vi "GetEnumValueAndPosition__slk_mt.vi"(7 "create enum configure":T1, 8 "error in (no error)":errorcluster, 11 "selection list":refnum<vi>[](array[refnum])) -> (0 "error out":errorcluster, 2 "position":cluster{"Left":i32, "Top":i32}, 3 "values":string[](array[string]), 4 "not found?":bool)   [LabVIEW 2013, in "Lazyboots Menu Tool.lvlib"]
doc: "Returns enum value and position."
uses:
  Library/Lazyboots Menu Tool.lvlib
  <vilib>/Utility/miscctls.llb/LVPositionTypeDef.ctl
  TypeDef/TypeDef_CreateEnumConfigure__slk_mt.ctl
panel:
  # "GetEnumValueAndPosition__slk_mt.vi\nReturns enum value and position.\n\nNOTICE -- YOU MUST LEAVE THIS NOTICE IN PLACE.\n\nCopyright (c) 2011, LIANG LIU Shawn.Liu.cn@gmail.com\nAll rights reserved.\n\nRedistribution and use in source and binary forms, with or without modification, are permitted provided that the following conditions are met:\n-Redistributions of source code must retain the above copyright notice, this list of conditions and the following disclaimer.\n-Redistributions in binary form must reproduce the above copyright notice, this list of conditions and the following disclaimer in the documentation and/or other materials provided with the distribution.\n-Neither the name of the eLp nor the names of its contributors may be used to endorse or promote products derived from this software without specific prior written permission.\n\nTHIS SOFTWARE IS PROVIDED BY THE COPYRIGHT HOLDERS AND CONTRIBUTORS \"AS IS\" AND ANY EXPRESS OR IMPLIED WARRANTIES, INCLUDING, BUT NOT LIMITED TO, THE IMPLIED WARRANTIES OF MERCHANTABILITY AND FITNESS FOR A PARTICULAR PURPOSE ARE DISCLAIMED. IN NO EVENT SHALL THE COPYRIGHT HOLDER OR CONTRIBUTORS BE LIABLE FOR ANY DIRECT, INDIRECT, INCIDENTAL, SPECIAL, EXEMPLARY, OR CONSEQUENTIAL DAMAGES (INCLUDING, BUT NOT LIMITED TO, PROCUREMENT OF SUBSTITUTE GOODS OR SERVICES; LOSS OF USE, DATA, OR PROFITS; OR BUSINESS INTERRUPTION) HOWEVER CAUSED AND ON ANY THEORY OF LIABILITY, WHETHER IN CONTRACT, STRICT LIABILITY, OR TORT (INCLUDING NEGLIGENCE OR OTHERWISE) ARISING IN ANY WAY OUT OF THE USE OF THIS SOFTWARE, EVEN IF ADVISED OF THE POSSIBILITY OF SUCH DAMAGE."
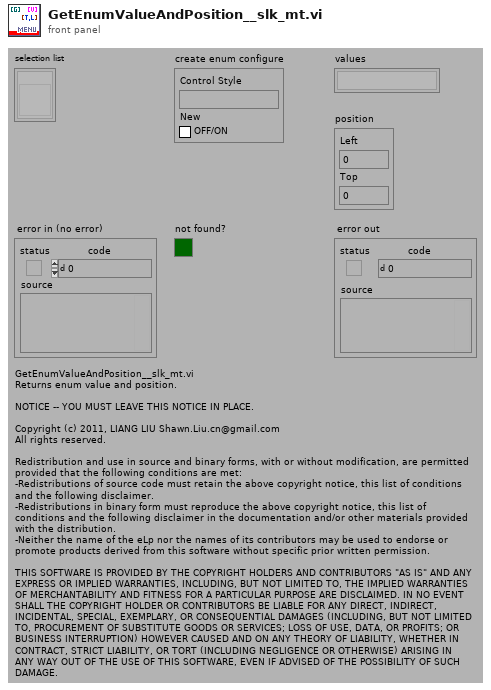
[diagram p1: front panel]
types:
  T1 = typedef "Lazyboots Menu Tool.lvlib/TypeDef_CreateEnumConfigure__slk_mt.ctl" = cluster{"Control Style":string, "New":bool}
  T2 = typedef "LVPositionTypeDef.ctl" = cluster{"Left":i32, "Top":i32}
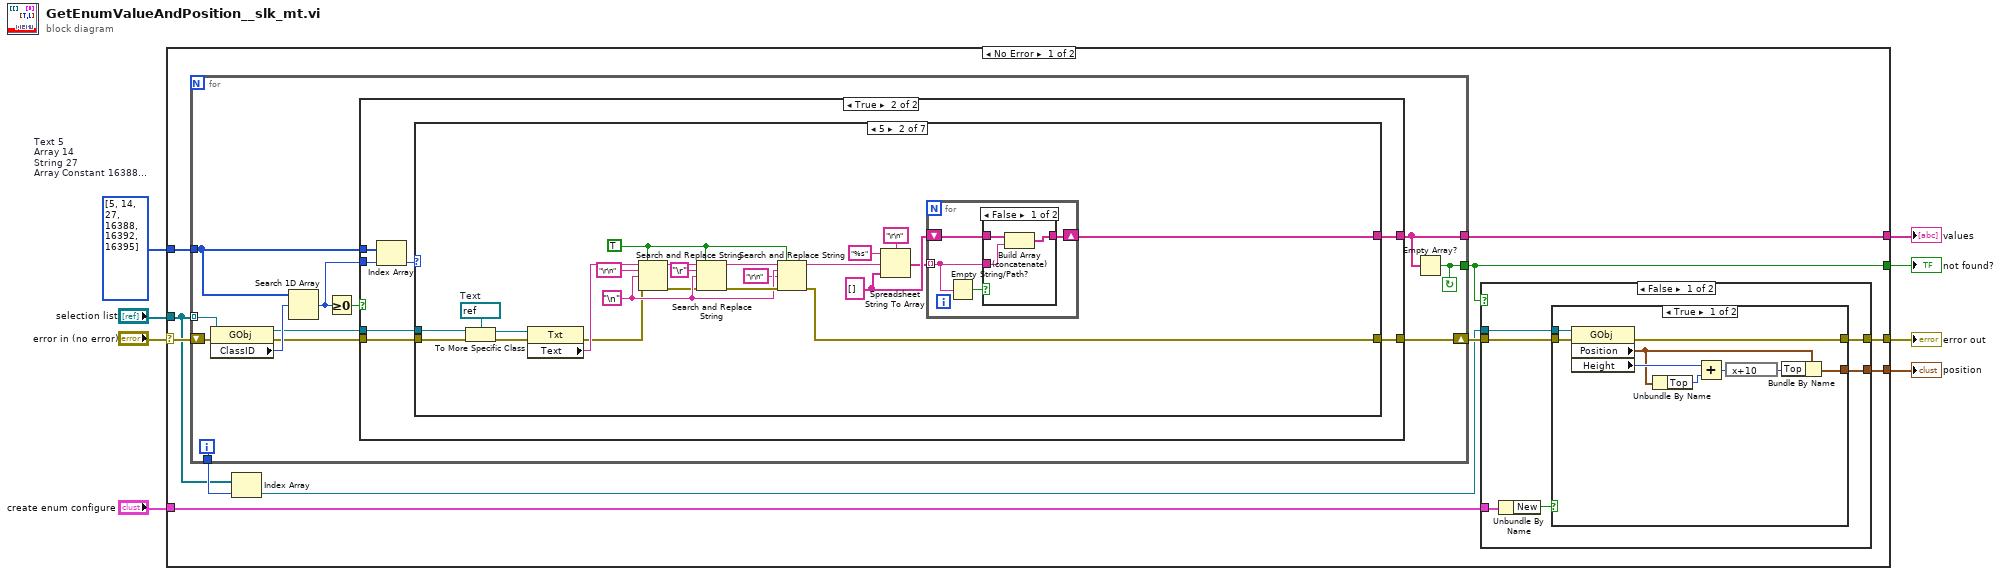
[diagram p0: block diagram]
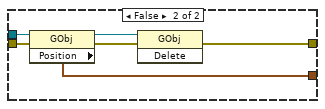
[diagram p2: hidden frame]
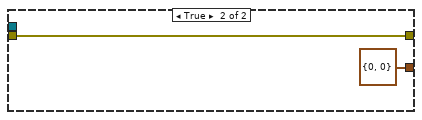
[diagram p3: hidden frame]
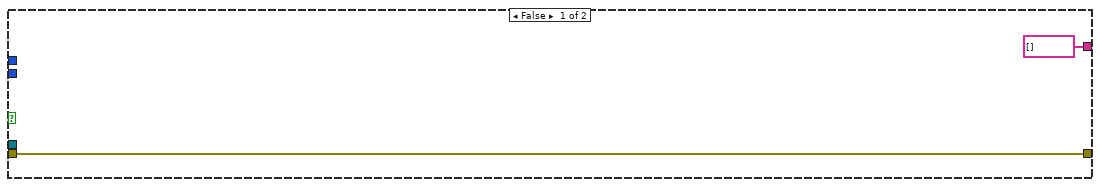
[diagram p4: hidden frame]
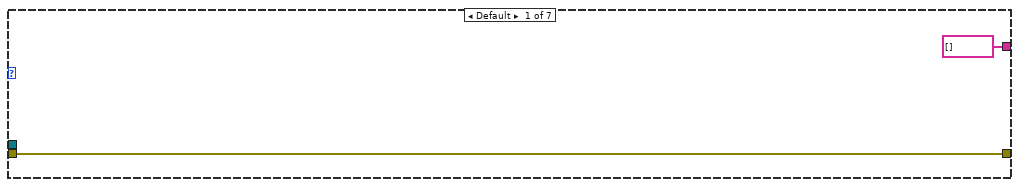
[diagram p5: hidden frame]
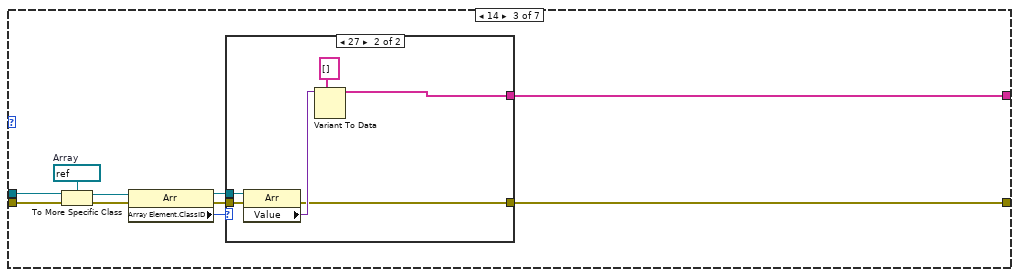
[diagram p7: hidden frame]
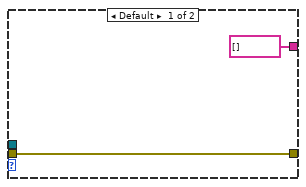
[diagram p8: hidden frame]
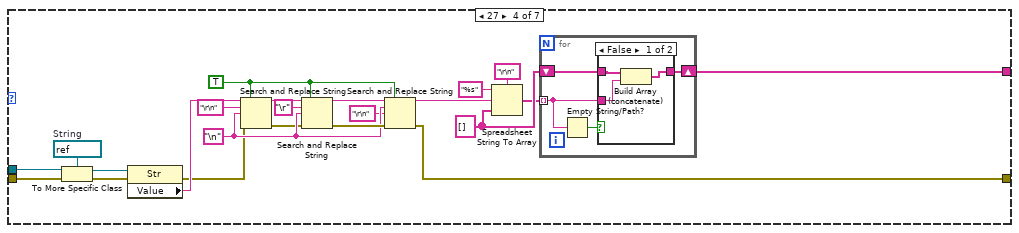
[diagram p9: hidden frame]
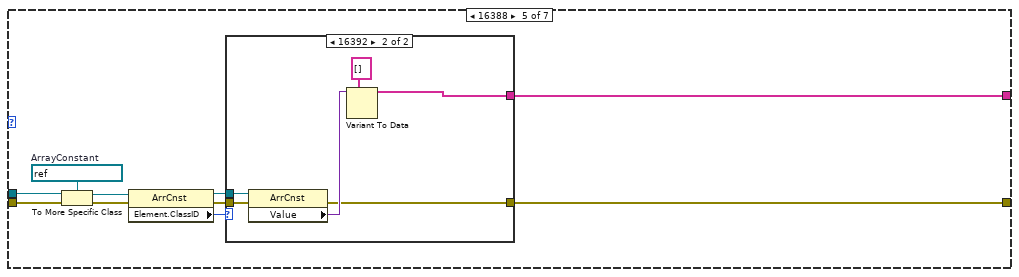
[diagram p11: hidden frame]
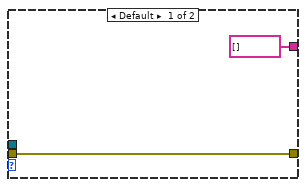
[diagram p12: hidden frame]
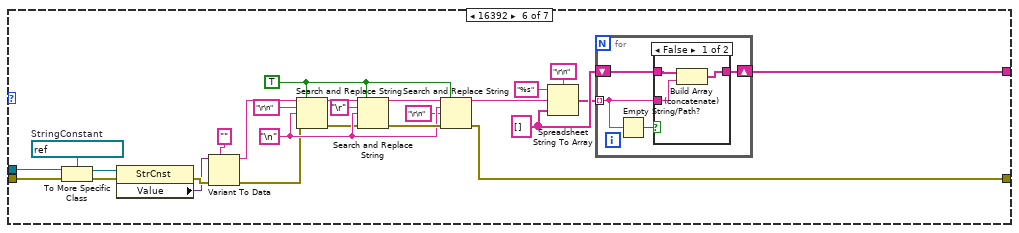
[diagram p13: hidden frame]
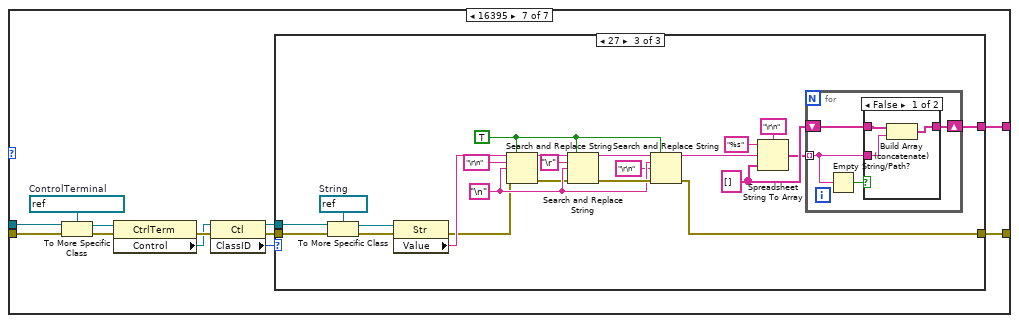
[diagram p15: hidden frame]
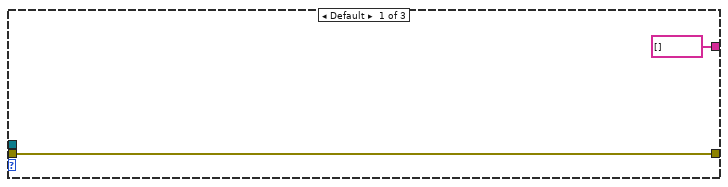
[diagram p16: hidden frame]
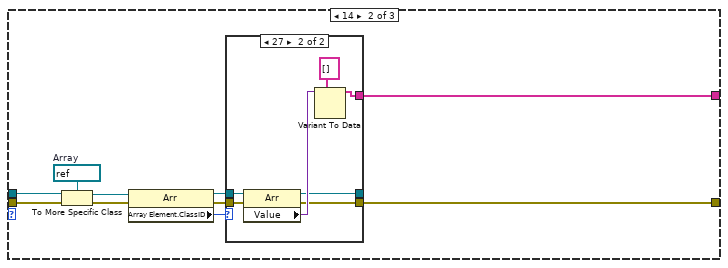
[diagram p17: hidden frame]
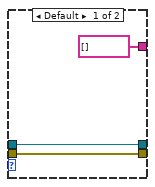
[diagram p18: hidden frame]
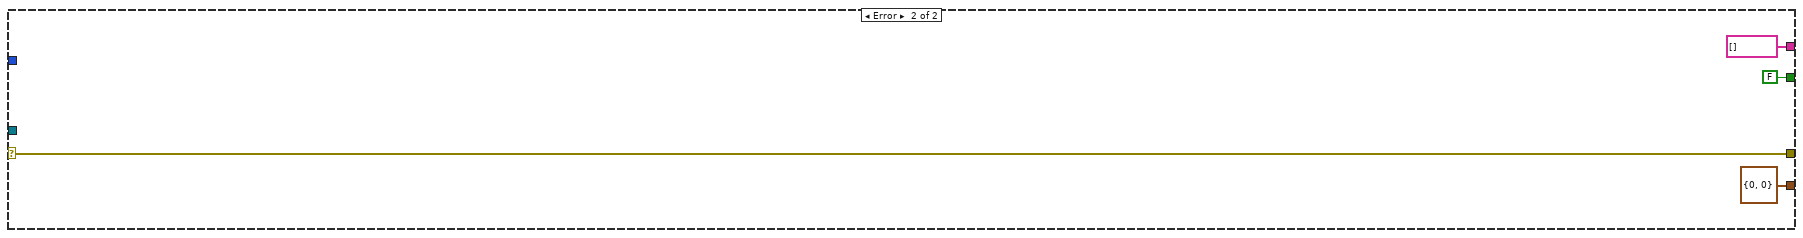
[diagram p20: hidden frame]
diagram:
  w8 = u32[] [5, 14, 27, 16388, 16392, 16395]  # Text 5 Array 14 String 27 Array Constant 16388 String Constant 16392 Control Terminal 16395
  n1 = case shown="No Error" "error in (no error)" {
    selector: "error in (no error)" -> [w17 w266]
    tunnel: w8 -> [w19 _]
    tunnel: [w18 string[] []] -> w7
    tunnel: "selection list" -> [w14 _]
    tunnel: [w12 FALSE ("empty?")] -> w4
    tunnel: [w11 w266] -> w3
    tunnel: [w10 T2 {"Left"=0, "Top"=0} ("Position")] -> w2
    tunnel: "create enum configure" -> [w9 _]
    frame No Error {
      n2 = for {
        tunnel: w19 -> [w53]
        tunnel: [w47] -> w18
        tunnel: w14 -> [w48] mode=indexing
        tunnel: [w46] -> w12
        shift-right: [w45] -> w16
        shift-left: w17 -> [w44]
        tunnel: [w43] -> w15
        i -> [w43]
        stop <- w46 continue-if-true
        n3 = property class="GObj"(reference=w48, error in=w44) -> (reference out=w50:refnum<vi>, error out=w49:errorcluster, "ClassID"=w54:u32)
        n4 = Search 1D Array(1D array=w53, element=w54) -> (index of element=w51:i32)  [unwired: 1 in]
        n5 = Greater Or Equal To 0?(x=w51) -> (x >= 0?=w52:bool)
        n6 = case shown="True" w52 {
          tunnel: w53 -> [_ w63]
          tunnel: w51 -> [_ w62]
          tunnel: w50 -> [_ w59]
          tunnel: w49 -> [w56 w60]
          tunnel: [w56 w57] -> w45
          tunnel: [string[] [] w58] -> w47
          frame False {
          }
          frame True {
            n7 = Index Array(array=w63, index=w62) -> (element=w61:u32)
            n8 = case shown="5" w61 {
              tunnel: w60 -> [w64 w70 w105 w119 w154 w172 w207]
              tunnel: w59 -> [_ w69 w104 w118 w153 w171 w206]
              tunnel: [w64 w67 w99 w116 w148 w169 w200] -> w57
              tunnel: [string[] [] w66 w100 w115 w149 w168 w199] -> w58
              frame Default {
              }
              frame 5 {
                w82 = string[] []
                w86 = "\n" ("search string")
                w88 = TRUE ("replace all? (F)")
                w71 = refnum<vi> refnum  # Text
                n9 = To More Specific Class(target class=w71, reference=w69, error in=w70) -> (specific class reference=w73:refnum<vi>, error out=w72:errorcluster)
                n10 = property class="Txt"(reference=w73, error in=w72) -> (error out=w68:errorcluster, "Text"=w77:string)  [unwired: 1 out]
                n11 = Search and Replace String(replace all?=w88, input string=w77, search string="\r\n", replace string=w86, error in=w68) -> (result string=w76:string, error out=w78:errorcluster)  [unwired: 5 out]
                n12 = Search and Replace String(replace all?=w88, input string=w76, search string="\r", replace string=w86, error in=w78) -> (result string=w85:string, error out=w87:errorcluster)  [unwired: 5 out]
                n13 = Search and Replace String(replace all?=w88, input string=w85, search string=w86, replace string="\r\n" ("replace string (\"\")"), error in=w87) -> (result string=w84:string, error out=w67:errorcluster)  [unwired: 3 in, 2 out]
                n14 = Spreadsheet String To Array(delimiter (Tab)="\r\n" ("search string"), format string="%s", spreadsheet string=w84, array type (2D Dbl)=w82) -> (array=w81:string[])
                n15 = for {
                  tunnel: w81 -> [w91] mode=indexing
                  shift-right: [w89] -> w66
                  shift-left: w82 -> [w90]
                  n16 = Empty String/Path?(string/path=w91) -> (empty?=w92:bool)
                  n17 = case shown="False" w92 {
                    tunnel: w91 -> [w93 _]
                    tunnel: w90 -> [w95 w96]
                    tunnel: [w94 w96] -> w89
                    frame False {
                      n18 = Build Array (concatenate)(w95, w93) -> (w94:string[])
                    }
                    frame True {
                    }
                  }
                }
              }
              frame 14 {
                w106 = refnum<vi> refnum  # Array
                n19 = To More Specific Class(target class=w106, reference=w104, error in=w105) -> (specific class reference=w101:refnum<vi>, error out=w102:errorcluster)
                n20 = property class="Arr"(reference=w101, error in=w102) -> (reference out=w98:refnum<vi>, error out=w97:errorcluster, "Array Element.ClassID"=w103:u32)
                n21 = case shown="27" w103 {
                  tunnel: [w108 w111] -> w99
                  tunnel: [string[] [] w112] -> w100
                  tunnel: w98 -> [_ w110]
                  tunnel: w97 -> [w108 w109]
                  frame Default {
                  }
                  frame 27 {
                    n22 = property class="Arr"(reference=w110, error in=w109) -> (error out=w111:errorcluster, "Value"=w114:variant)  [unwired: 1 out]
                    n23 = Variant To Data(type=string[] [], Variant=w114) -> (data=w112:string[])  [unwired: 1 in, 1 out]
                  }
                }
              }
              frame 27 {
                w131 = string[] []
                w135 = "\n" ("search string")
                w137 = TRUE ("replace all? (F)")
                w120 = refnum<vi> refnum  # String
                n24 = To More Specific Class(target class=w120, reference=w118, error in=w119) -> (specific class reference=w122:refnum<vi>, error out=w121:errorcluster)
                n25 = property class="Str"(reference=w122, error in=w121) -> (error out=w117:errorcluster, "Value"=w126:string)  [unwired: 1 out]
                n26 = Search and Replace String(replace all?=w137, input string=w126, search string="\r\n", replace string=w135, error in=w117) -> (result string=w125:string, error out=w127:errorcluster)  [unwired: 5 out]
                n27 = Search and Replace String(replace all?=w137, input string=w125, search string="\r", replace string=w135, error in=w127) -> (result string=w134:string, error out=w136:errorcluster)  [unwired: 5 out]
                n28 = Search and Replace String(replace all?=w137, input string=w134, search string=w135, replace string="\r\n" ("replace string (\"\")"), error in=w136) -> (result string=w133:string, error out=w116:errorcluster)  [unwired: 3 in, 2 out]
                n29 = Spreadsheet String To Array(delimiter (Tab)="\r\n" ("search string"), format string="%s", spreadsheet string=w133, array type (2D Dbl)=w131) -> (array=w130:string[])
                n30 = for {
                  tunnel: w130 -> [w140] mode=indexing
                  shift-right: [w138] -> w115
                  shift-left: w131 -> [w139]
                  n31 = Empty String/Path?(string/path=w140) -> (empty?=w141:bool)
                  n32 = case shown="False" w141 {
                    tunnel: w140 -> [w142 _]
                    tunnel: w139 -> [w144 w145]
                    tunnel: [w143 w145] -> w138
                    frame False {
                      n33 = Build Array (concatenate)(w144, w142) -> (w143:string[])
                    }
                    frame True {
                    }
                  }
                }
              }
              frame 16388 {
                w155 = refnum<vi> refnum  # ArrayConstant
                n34 = To More Specific Class(target class=w155, reference=w153, error in=w154) -> (specific class reference=w150:refnum<vi>, error out=w151:errorcluster)
                n35 = property class="ArrCnst"(reference=w150, error in=w151) -> (reference out=w147:refnum<vi>, error out=w146:errorcluster, "Element.ClassID"=w152:u32)
                n36 = case shown="16392" w152 {
                  tunnel: [w157 w160] -> w148
                  tunnel: [string[] [] w161] -> w149
                  tunnel: w147 -> [_ w159]
                  tunnel: w146 -> [w157 w158]
                  frame Default {
                  }
                  frame 16392 {
                    n37 = property class="ArrCnst"(reference=w159, error in=w158) -> (error out=w160:errorcluster, "Value"=w163:variant)  [unwired: 1 out]
                    n38 = Variant To Data(type=string[] [], Variant=w163) -> (data=w161:string[])  [unwired: 1 in, 1 out]
                  }
                }
              }
              frame 16392 {
                w183 = string[] []
                w187 = "\n" ("search string")
                w189 = TRUE ("replace all? (F)")
                w173 = refnum<vi> refnum  # StringConstant
                n39 = To More Specific Class(target class=w173, reference=w171, error in=w172) -> (specific class reference=w175:refnum<vi>, error out=w174:errorcluster)
                n40 = property class="StrCnst"(reference=w175, error in=w174) -> (error out=w170:errorcluster, "Value"=w166:variant)  [unwired: 1 out]
                n41 = Variant To Data(error in=w170, type="", Variant=w166) -> (data=w165:string, error out=w167:errorcluster)
                n42 = Search and Replace String(replace all?=w189, input string=w165, search string="\r\n", replace string=w187, error in=w167) -> (result string=w178:string, error out=w179:errorcluster)  [unwired: 5 out]
                n43 = Search and Replace String(replace all?=w189, input string=w178, search string="\r", replace string=w187, error in=w179) -> (result string=w186:string, error out=w188:errorcluster)  [unwired: 5 out]
                n44 = Search and Replace String(replace all?=w189, input string=w186, search string=w187, replace string="\r\n" ("replace string (\"\")"), error in=w188) -> (result string=w185:string, error out=w169:errorcluster)  [unwired: 3 in, 2 out]
                n45 = Spreadsheet String To Array(delimiter (Tab)="\r\n" ("search string"), format string="%s", spreadsheet string=w185, array type (2D Dbl)=w183) -> (array=w182:string[])
                n46 = for {
                  tunnel: w182 -> [w192] mode=indexing
                  shift-right: [w190] -> w168
                  shift-left: w183 -> [w191]
                  n47 = Empty String/Path?(string/path=w192) -> (empty?=w193:bool)
                  n48 = case shown="False" w193 {
                    tunnel: w192 -> [w194 _]
                    tunnel: w191 -> [w196 w197]
                    tunnel: [w195 w197] -> w190
                    frame False {
                      n49 = Build Array (concatenate)(w196, w194) -> (w195:string[])
                    }
                    frame True {
                    }
                  }
                }
              }
              frame 16395 {
                w208 = refnum<vi> refnum  # ControlTerminal
                n50 = To More Specific Class(target class=w208, reference=w206, error in=w207) -> (specific class reference=w198:refnum<vi>, error out=w209:errorcluster)
                n51 = property class="CtrlTerm"(reference=w198, error in=w209) -> (error out=w205:errorcluster, "Control"=w204:refnum<vi>)  [unwired: 1 out]
                n52 = property class="Ctl"(reference=w204, error in=w205) -> (reference out=w202:refnum<vi>, error out=w203:errorcluster, "ClassID"=w201:u32)
                n53 = case shown="27" w201 {
                  tunnel: w203 -> [w210 w220 w236]
                  tunnel: w202 -> [_ w219 w235]
                  tunnel: [w210 w214 w233] -> w200
                  tunnel: [string[] [] w215 w232] -> w199
                  frame Default {
                  }
                  frame 14 {
                    w221 = refnum<vi> refnum  # Array
                    n54 = To More Specific Class(target class=w221, reference=w219, error in=w220) -> (specific class reference=w216:refnum<vi>, error out=w217:errorcluster)
                    n55 = property class="Arr"(reference=w216, error in=w217) -> (reference out=w213:refnum<vi>, error out=w212:errorcluster, "Array Element.ClassID"=w218:u32)
                    n56 = case shown="27" w218 {
                      tunnel: [w224 w228] -> w214
                      tunnel: [string[] [] w229] -> w215
                      tunnel: [w223 w227] -> _
                      tunnel: w213 -> [w223 w226]
                      tunnel: w212 -> [w224 w225]
                      frame Default {
                      }
                      frame 27 {
                        n57 = property class="Arr"(reference=w226, error in=w225) -> (reference out=w227:refnum<vi>, error out=w228:errorcluster, "Value"=w231:variant)
                        n58 = Variant To Data(type=string[] [], Variant=w231) -> (data=w229:string[])  [unwired: 1 in, 1 out]
                      }
                    }
                  }
                  frame 27 {
                    w248 = string[] []
                    w252 = "\n" ("search string")
                    w254 = TRUE ("replace all? (F)")
                    w237 = refnum<vi> refnum  # String
                    n59 = To More Specific Class(target class=w237, reference=w235, error in=w236) -> (specific class reference=w239:refnum<vi>, error out=w238:errorcluster)
                    n60 = property class="Str"(reference=w239, error in=w238) -> (error out=w234:errorcluster, "Value"=w243:string)  [unwired: 1 out]
                    n61 = Search and Replace String(replace all?=w254, input string=w243, search string="\r\n", replace string=w252, error in=w234) -> (result string=w242:string, error out=w244:errorcluster)  [unwired: 5 out]
                    n62 = Search and Replace String(replace all?=w254, input string=w242, search string="\r", replace string=w252, error in=w244) -> (result string=w251:string, error out=w253:errorcluster)  [unwired: 5 out]
                    n63 = Search and Replace String(replace all?=w254, input string=w251, search string=w252, replace string="\r\n" ("replace string (\"\")"), error in=w253) -> (result string=w250:string, error out=w233:errorcluster)  [unwired: 3 in, 2 out]
                    n64 = Spreadsheet String To Array(delimiter (Tab)="\r\n" ("search string"), format string="%s", spreadsheet string=w250, array type (2D Dbl)=w248) -> (array=w247:string[])
                    n65 = for {
                      tunnel: w247 -> [w257] mode=indexing
                      shift-right: [w255] -> w232
                      shift-left: w248 -> [w256]
                      n66 = Empty String/Path?(string/path=w257) -> (empty?=w258:bool)
                      n67 = case shown="False" w258 {
                        tunnel: w257 -> [w259 _]
                        tunnel: w256 -> [w261 w262]
                        tunnel: [w260 w262] -> w255
                        frame False {
                          n68 = Build Array (concatenate)(w261, w259) -> (w260:string[])
                        }
                        frame True {
                        }
                      }
                    }
                  }
                }
              }
            }
          }
        }
        n69 = Empty Array?(array=w47) -> (empty?=w46:bool)
      }
      n70 = Index Array(array=w14, index=w15) -> (element=w13:refnum<vi>)
      n71 = case shown="False" w12 {
        tunnel: w16 -> [w25 w42]
        tunnel: w13 -> [w24 _]
        tunnel: [w23 w42] -> w11
        tunnel: [w22 T2 {"Left"=0, "Top"=0} ("Position")] -> w10
        tunnel: w9 -> [w20 _]
        frame False {
          n72 = Unbundle By Name(w20) -> ("New"=w21:bool)
          n73 = case shown="True" w21 {
            tunnel: [w31 w37] -> w23
            tunnel: [w30 w40] -> w22
            tunnel: w25 -> [w27 w36]
            tunnel: w24 -> [w26 w35]
            frame True {
              n74 = property class="GObj"(reference=w26, error in=w27) -> (error out=w31:errorcluster, "Position"=w29:T2, "Height"=w33:u32)  [unwired: 1 out]
              n75 = Unbundle By Name(w29) -> ("Top"=w32:i32)
              n76 = Add(x=w33, y=w32) -> (x+y=w34:u32)
              n77 = expression code="x+10"(w34) -> (w28:u32)
              n78 = Bundle By Name(cluster=w29, "Top"=w28) -> (w30:T2)
            }
            frame False {
              n79 = property class="GObj"(reference=w35, error in=w36) -> (reference out=w38:refnum<vi>, error out=w39:errorcluster, "Position"=w40:T2)
              n80 = invoke class="GObj" method="Delete"(reference=w38, error in=w39) -> (error out=w37:errorcluster)  [unwired: 1 in, 2 out]
            }
          }
        }
        frame True {
        }
      }
    }
    frame Error {
    }
  }
  "values" <- w7
  "position" <- w2
  "error out" <- w3
  "not found?" <- w4
